vi "FTW-Message-Initialize.vi"(0 "FTW Message":refnum<class "FTW-Message.lvclass">, 5 "Sender Identity":string, 7 "Message Header":string, 9 "Message Body":string, 11 "error in":errorcluster) -> (4 "FTW Message out":refnum<class "FTW-Message.lvclass">, 15 "error out":errorcluster)   [LabVIEW 2013, in "FTW-Actor.lvlib" / "FTW-Message.lvclass"]
uses:
  FTW-Message.lvclass
panel:
  # "Inputs"
  # "Outputs"
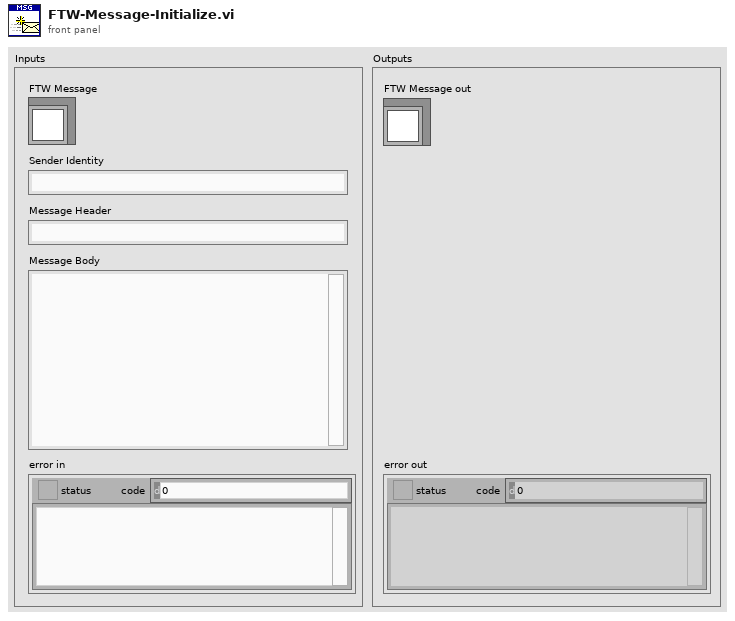
[diagram p1: front panel]
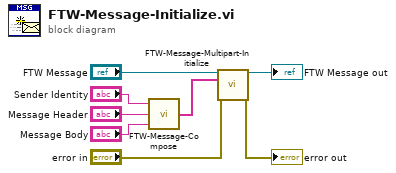
[diagram p0: block diagram]
diagram:
  n1 = call "FTW-Message-Compose.vi"("Message Body"="Message Body", "Message Header"="Message Header", "Sender Identity"="Sender Identity") -> ("Multipart Message"=w3:string[])  [unwired: 1 in]
  n2 = call-dynamic "FTW-Message-Multipart-Initialize.vi"("FTW Message"="FTW Message", "Message Parts"=w3, "error in"="error in") -> ("FTW Message out"=→"FTW Message out":refnum<class "FTW-Message.lvclass">, "error out"=→"error out":errorcluster)  [unwired: 11 in]
